vi "CSConnect.CalculateVoltages.vi"(0 "i ref in":refnum<vi>, 5 "error in (no error)":errorcluster) -> (14 "i ref out":refnum<vi>, 16 "Array Out-Voltages":dbl[](array[numeric]), 19 "error out":errorcluster)   [LabVIEW 2014, in "CSConnect.lvlib"]
doc: "Calculates the voltage of a channel.\n\nLicense Agreement for this software:\n\nCopyright (C)\nGesellschaft für Schwerionenforschung, GSI\nPlanckstr. 1\n64291 Darmstadt\nGermany\n\nContact: D.Beck@gsi.de \n\nThis program is free software; you can redistribute it and/or modify it under the terms of the \nGNU General Public License as published by the Free Software Foundation; either version 2 of \nthe license, or (at your option) any later version.\n\nThis program is distributed in the hope that it will be useful, but WITHOUT ANY WARRANTY; \nwithout even the implied warranty of MERCHANTABILITY or FITNESS FOR A PARTICULAR PURPOSE. See the GNU General License for more details (http://www.gnu.org).\n\nGesellschaft für Schwerionenforschung, GSI\nPlanckstr. 1, 64291 Darmstadt, Germany\nFor all questions and ideas contact: M.Richter@gsi.de, H.Brand@gsi.de or D.Beck@gsi.de.\nLast update: 16-JUN-2004"
uses:
  CSConnect.lvlib
  <vilib>/gmath/NI_Gmath.lvlib
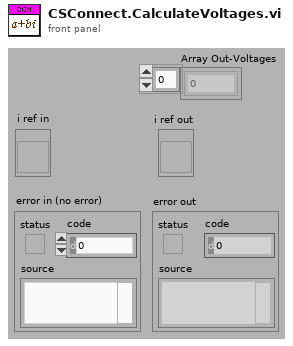
[diagram p1: front panel]
types:
  T1 = typedef "CSConnect.lvlib/CSConnect.i attribute.ctl" = cluster{"In-Array":cluster{"Alias":string, "Value":dbl, "neededOuts":bool[]}[], "Out-Array":cluster{"ObjectName":string, "VoltFunctionName":string, "OnOffFunctionName":string, "Channel":string, "Calculation-Formula":string}[], "OutChannelsID":i32, "InOutMatrixID":i32}
  T2 = cluster{"ObjectName":string, "VoltFunctionName":string, "OnOffFunctionName":string, "Channel":string, "Calculation-Formula":string}[]
  T3 = cluster{"Alias":string, "Value":dbl, "neededOuts":bool[]}[]
  T4 = cluster{"ObjectName":string, "VoltFunctionName":string, "OnOffFunctionName":string, "Channel":string, "Calculation-Formula":string}
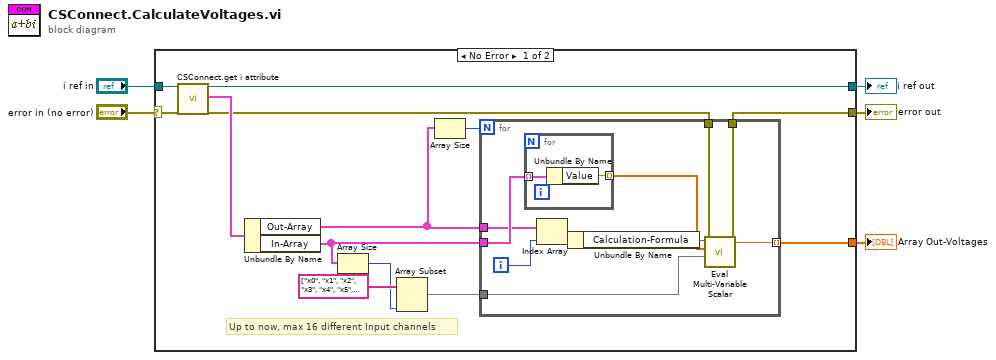
[diagram p0: block diagram]
diagram:
  n1 = case shown="No Error" "error in (no error)" {
    selector: "error in (no error)" -> [w17 w31]
    tunnel: [w15 w31] -> w5
    tunnel: [w13 w32] -> w3
    tunnel: "i ref in" -> [w18 w32]
    tunnel: [w12 _] -> w1
    frame No Error {
      # "Up to now, max 16 different Input channels"
      n2 = call "CSConnect.get i attribute.vi"("i ref in"=w18, "error in (no error)"=w17) -> ("i ref out"=w13:refnum<vi>, "i attribute"=w16:T1, "error out"=w14:errorcluster)  [unwired: 15 in]
      n3 = Unbundle By Name(w16) -> ("Out-Array"=w11:T2, "In-Array"=w9:T3)
      n4 = Array Size(array=w9) -> (size(s)=w7:i32)
      n5 = Array Subset(array=string[] ["x0", "x1", "x2", "x3", "x4", "x5", "x6", "x7", "x8", "x9", "x10", "x11", "x12", "x13", "x14", "x15"] ("Variables"), length=w7) -> (w6:string[])  [unwired: 1 in]
      n6 = Array Size(array=w11) -> (size(s)=w10:i32)
      n7 = for {
        N: w10 -> [_]
        tunnel: w9 -> [w26]
        tunnel: [w24] -> w15
        tunnel: w14 -> [w23]
        tunnel: [w22] -> w12 mode=indexing
        tunnel: w11 -> [w21]
        tunnel: w6 -> [w19]
        i -> [w20]
        n8 = for {
          tunnel: w26 -> [w30] mode=indexing
          tunnel: [w29] -> w25 mode=indexing
          n9 = Unbundle By Name(w30) -> ("Value"=w29:dbl)
        }
        n10 = Index Array(array=w21, index=w20) -> (element=w28:T4)
        n11 = Unbundle By Name(w28) -> ("Calculation-Formula"=w27:string)
        n12 = call <vilib>:"Eval Multi-Variable Scalar.vi"("error in (no error)"=w23, "Variables"=w19, "X Values"=w25, "formula"=w27) -> ("error out"=w24:errorcluster, "y value"=w22:dbl)
      }
    }
    frame Error {
    }
  }
  "error out" <- w5
  "i ref out" <- w3
  "Array Out-Voltages" <- w1
